vi "StartTest.vi"(7 "LabVIEW Web Service Request":refnum<class "Web Request.lvclass">) -> ()   [LabVIEW 2014]
uses:
  <vilib>/wsapi/Web Request.lvclass
  Coding Platform.lvlib
panel:
  # "Use the Web Service Request input terminal to call the VIs on the Web Services palette. Do not remove it from the connector pane unless you don't need access to the palette."
  # "Each additional control wired to the connector pane will be available as an input in the URL. To include an indicator in terminal-mode output (the default setting), it must also be wired to the connector pane."
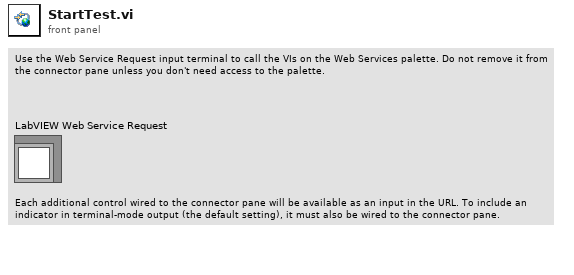
[diagram p1: front panel]
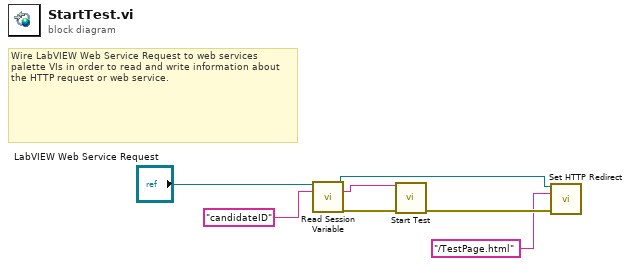
[diagram p0: block diagram]
diagram:
  # "Wire LabVIEW Web Service Request to web services palette VIs in order to read and write information about the HTTP request or web service."
  n1 = call <vilib>:"Read Session Variable.vi"("LabVIEW Web Service Request"="LabVIEW Web Service Request", "key"="candidateID") -> ("LabVIEW Web Service Request out"=w2:refnum<class "Web Request.lvclass">, "value"=w4:string, "error out"=w5:errorcluster)  [unwired: 11 in]
  n2 = call "Start Test.vi"("Candidate ID"=w4, "error in (no error)"=w5) -> ("error out"=w3:errorcluster)  [unwired: 12 in, 1 out]
  n3 = call <vilib>:"Set HTTP Redirect.vi"("LabVIEW Web Service Request"=w2, "redirect URL"="/TestPage.html", "error in (no error)"=w3) -> ()  [unwired: 11 in, 2 out]
